vi "Cartesian to Polar.vi"(8 "Y":dbl, 11 "Z":dbl) -> (0 "Phi":dbl, 3 "B":dbl)   [LabVIEW 2019]
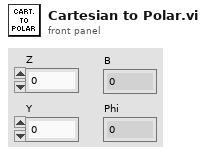
[diagram p1: front panel]
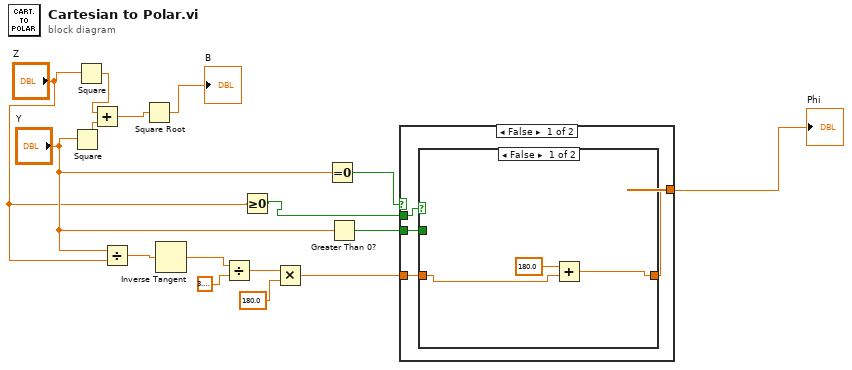
[diagram p0: block diagram]
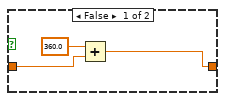
[diagram p3: hidden frame]
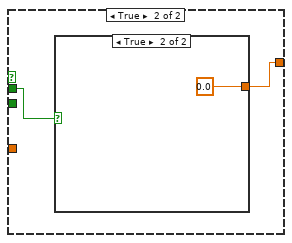
[diagram p4: hidden frame]
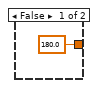
[diagram p5: hidden frame]
diagram:
  n1 = Square(x="Y") -> (x^2=w15:dbl)
  n2 = Square(x="Z") -> (x^2=w16:dbl)
  n3 = Add(x=w16, y=w15) -> (x+y=w14:dbl)
  n4 = Divide(x="Y", y="Z") -> (x/y=w12:dbl)
  n5 = Square Root(x=w14) -> (sqrt(x)=→"B":dbl)
  n6 = Inverse Tangent(1:w12) -> (0:w11:dbl)
  n7 = Divide(x=w11, y=3.141592653589793) -> (x/y=w9:dbl)
  n8 = Greater Or Equal To 0?(x="Z") -> (x >= 0?=w2:bool)
  n9 = Multiply(x=w9, y=180.0) -> (x*y=w3:dbl)
  n10 = Equal To 0?(x="Y") -> (x = 0?=w7:bool)
  n11 = Greater Than 0?(x="Y") -> (x > 0?=w4:bool)
  n12 = case shown="False" w7 {
    tunnel: [w17 w31] -> w6
    tunnel: w2 -> [w20 w32]
    tunnel: w4 -> [w19 _]
    tunnel: w3 -> [w18 _]
    frame False {
      n13 = case shown="False" w20 {
        tunnel: w19 -> [_ w26]
        tunnel: w18 -> [w22 w24]
        tunnel: [w21 w25] -> w17
        frame False {
          n14 = Add(x=180.0, y=w22) -> (x+y=w21:dbl)
        }
        frame True {
          n15 = case shown="True" w26 {
            tunnel: [w27 w30] -> w25
            tunnel: w24 -> [w28 w30]
            frame False {
              n16 = Add(x=360.0, y=w28) -> (x+y=w27:dbl)
            }
            frame True {
            }
          }
        }
      }
    }
    frame True {
      n17 = case shown="True" w32 {
        tunnel: [180.0 0.0] -> w31
        frame False {
        }
        frame True {
        }
      }
    }
  }
  "Phi" <- w6
